vi "End.vi"(8 "error in (no error)":errorcluster, 11 "S4ACS_GUI in":refnum<class "S4ACS_GUI.lvclass">) -> (0 "error out":errorcluster, 3 "S4ACS_GUI out":refnum<class "S4ACS_GUI.lvclass">)   [LabVIEW 2012, in "S4ACS_GUI.lvclass"]
uses:
  S4ACS_GUI.lvclass
  S4ACS_GUI.lvclass/S4ACS_GUI.ctl
  Acquisition/Acquisition.lvclass
  SyncBox/Sync Box.lvclass
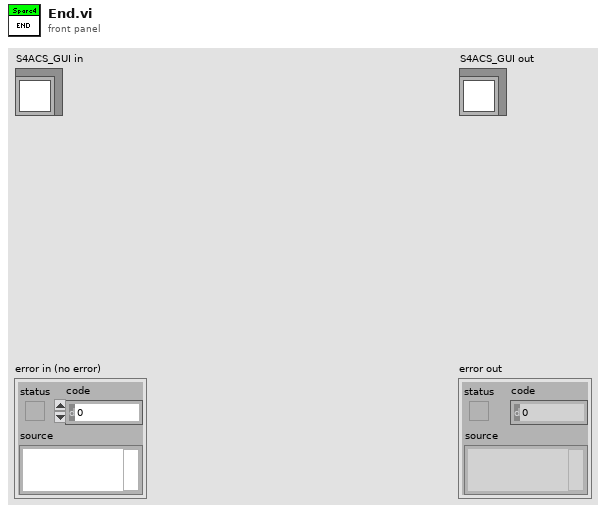
[diagram p1: front panel]
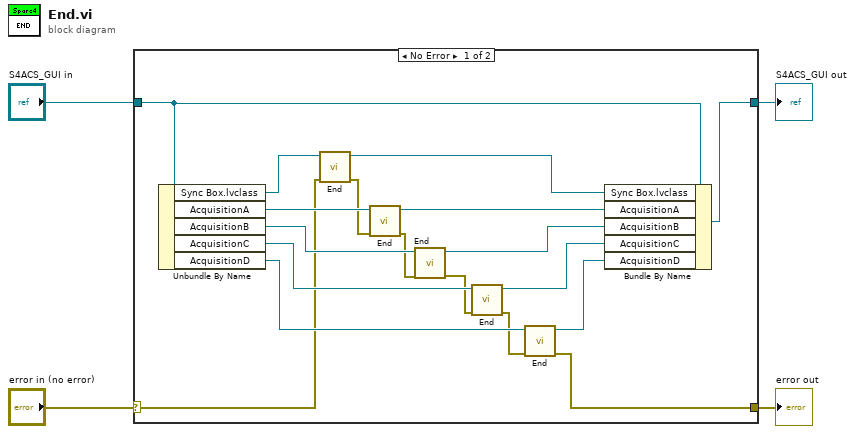
[diagram p0: block diagram]
diagram:
  n1 = case shown="No Error" "error in (no error)" {
    selector: "error in (no error)" -> [w6 w24]
    tunnel: [w9 w24] -> w3
    tunnel: [w18 w23] -> w1
    tunnel: "S4ACS_GUI in" -> [w19 w23]
    frame No Error {
      n2 = Unbundle By Name(w19) -> ("Sync Box.lvclass"=w8:refnum<class "Sync Box.lvclass">, "AcquisitionA"=w22:refnum<class "Acquisition.lvclass">, "AcquisitionB"=w21:refnum<class "Acquisition.lvclass">, "AcquisitionC"=w17:refnum<class "Acquisition.lvclass">, "AcquisitionD"=w20:refnum<class "Acquisition.lvclass">)
      n3 = call "End.vi"("error in (no error)"=w6, "Sync Box in"=w8) -> ("error out"=w5:errorcluster, "Sync Box out"=w7:refnum<class "Sync Box.lvclass">)  [unwired: 8 in]
      n4 = call-dynamic "End.vi"("error in (no error)"=w5, "Acquisition in"=w22) -> ("error out"=w15:errorcluster, "Acquisition out"=w13:refnum<class "Acquisition.lvclass">)  [unwired: 8 in]
      n5 = call-dynamic "End.vi"("error in (no error)"=w15, "Acquisition in"=w21) -> ("error out"=w16:errorcluster, "Acquisition out"=w12:refnum<class "Acquisition.lvclass">)  [unwired: 8 in]
      n6 = call-dynamic "End.vi"("error in (no error)"=w16, "Acquisition in"=w17) -> ("error out"=w14:errorcluster, "Acquisition out"=w11:refnum<class "Acquisition.lvclass">)  [unwired: 8 in]
      n7 = call-dynamic "End.vi"("error in (no error)"=w14, "Acquisition in"=w20) -> ("error out"=w9:errorcluster, "Acquisition out"=w10:refnum<class "Acquisition.lvclass">)  [unwired: 8 in]
      n8 = Bundle By Name(cluster=w19, "Sync Box.lvclass"=w7, "AcquisitionA"=w13, "AcquisitionB"=w12, "AcquisitionC"=w11, "AcquisitionD"=w10) -> (w18:refnum<class "S4ACS_GUI.lvclass">)
    }
    frame Error {
    }
  }
  "error out" <- w3
  "S4ACS_GUI out" <- w1
